vi "Codec_CMD_25.vi"(8 "error in (no error)":errorcluster, 10 "AskCMD25":T1={"STATION"="H/P", "RACK"="1", "DUT"="1"}, 11 "SecureMqttCodec in":refnum<class "SecureMqttCodec.lvclass">) -> (0 "error out":errorcluster, 2 "<JSON>":string="{\r  \"CMD\": 25,\r  \"CONTENT\": [\r    {\r      \"DUT\": \"1\",\r      \"RACK\": \"1\",\r      \"STATION\": \"H/P\"\r    }\r  ],\r  \"ERRCODE\": \"\",\r  \"ERRMSG\": \"\",\r  \"FROM\": \"845CF3525B43\",\r  \"ID\": \"BEEA132C-7671-42B7-B8AF-0AE4588F97BB\",\r  \"STATUS\": \"\",\r  \"TIMESTAMP\": 1759592435,\r  \"TO\": \"\"\r}", 3 "SecureMqttCodec out":refnum<class "SecureMqttCodec.lvclass">)   [LabVIEW 2020, in "SecureMqttCodec.lvclass"]
uses:
  SecureMqttCodec.lvclass
  TestMQTT/Ctrl/ReplyCMD25.ctl
  SecureMqttCodec.lvclass/SecureMqttCodec.ctl
  <vilib>/addons/JSON API/JSON Value/Set from JSON string.vi
  <vilib>/addons/JSON API/JSON Scalar/JSON Scalar.lvclass
  C:/Program Files/National Instruments/LabVIEW 2020/vi.lib/addons/JSON API/JSON Value/JSON Value.lvclass
  <vilib>/addons/JSON API/JSON Array/JSON Array.lvclass
  <vilib>/addons/JSON API/JSON Scalar/Set U32.vi
  <vilib>/addons/JSON API/JSON Array/Set JSON Array.vi
  <vilib>/addons/JSON API/JSON Value/Get as JSON string (pretty).vi
  <vilib>/addons/JSON API/JSON Value/JSON Value.lvclass
  <vilib>/addons/JSON API/Get Polymorphic/JSON GetSet.lvlib
  <vilib>/addons/JSON API/JSON Object/JSON Object.lvclass
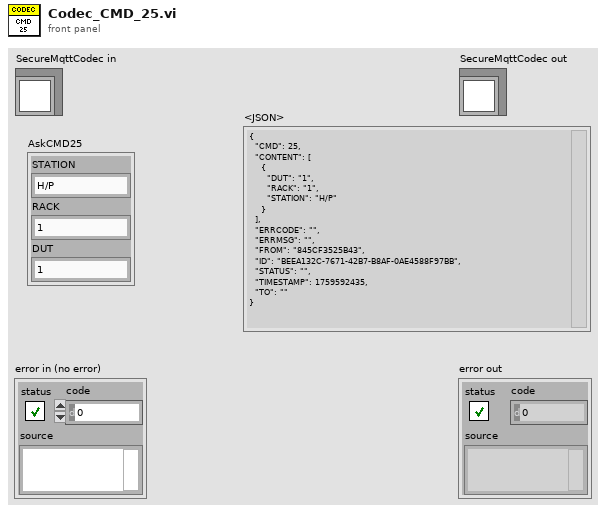
[diagram p1: front panel]
types:
  T1 = typedef "ReplyCMD25.ctl" = cluster{"STATION":string, "RACK":string, "DUT":string}
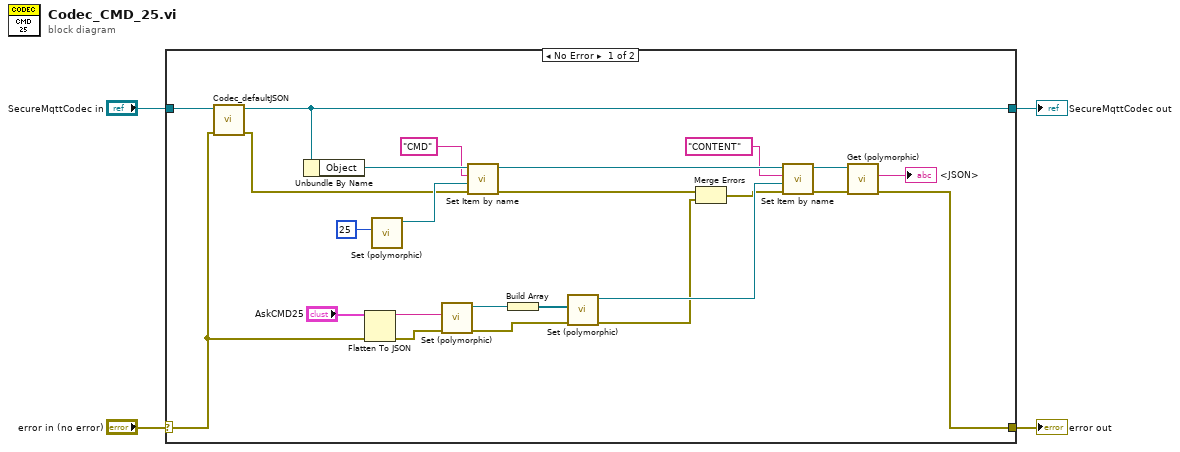
[diagram p0: block diagram]
diagram:
  n1 = case shown="No Error" "error in (no error)" {
    selector: "error in (no error)" -> [w8 w30]
    tunnel: [w24 w30] -> w3
    tunnel: [w16 w29] -> w1
    tunnel: "SecureMqttCodec in" -> [w28 w29]
    frame No Error {
      n2 = call "Codec_defaultJSON.vi"("error in (no error)"=w8, "SecureMqttCodec in"=w28) -> ("error out"=w15:errorcluster, "SecureMqttCodec out"=w16:refnum<class "SecureMqttCodec.lvclass">)  [unwired: 8 in]
      n3 = Unbundle By Name(w16) -> ("Object"=w27:refnum<class "JSON Value.lvclass">)
      n4 = Flatten To JSON(anything="AskCMD25", error in (no error)=w8) -> (JSON string=w10:string, 11:w9:errorcluster)  [unwired: 1 in]
      n5 = call-poly <vilib>:"Set (polymorphic).vi"("Numeric"=u32 25) -> ("JSON Scalar out"=w25:refnum<class "JSON Scalar.lvclass">)  [unwired: 9 in, 1 out]
      n6 = call-poly <vilib>:"Set (polymorphic).vi"("error in (no error)"=w9, "JSON stream"=w10) -> ("error out"=w7:errorcluster, "JSON Value out"=w12:refnum<class "JSON Value.lvclass">)  [unwired: 7 in, 1 out]
      n7 = call-dynamic "Set Item by name.vi"("error in (no error)"=w15, "Value"=w25, "name"="CMD", "JSON Value In"=w27) -> ("error out"=w20:errorcluster, "JSON Value Out"=w22:refnum<class "JSON Value.lvclass">)  [unwired: 5 in, 1 out]
      n8 = Build Array(w12) -> (w11:refnum<class "JSON Value.lvclass">[])
      n9 = call-poly <vilib>:"Set (polymorphic).vi"("error in (no error)"=w7, "Array"=w11) -> ("error out"=w5:errorcluster, "JSON Array out"=w18:refnum<class "JSON Array.lvclass">)  [unwired: 8 in]
      n10 = Merge Errors(w20, w5) -> (w6:errorcluster)
      n11 = call-dynamic "Set Item by name.vi"("error in (no error)"=w6, "Value"=w18, "name"="CONTENT", "JSON Value In"=w22) -> ("error out"=w19:errorcluster, "JSON Value Out"=w21:refnum<class "JSON Value.lvclass">)  [unwired: 5 in, 1 out]
      n12 = call-poly <vilib>:"Get (polymorphic).vi"("error in (no error)"=w19, "JSON Value in"=w21) -> ("error out"=w24:errorcluster, "<JSON>"=→"<JSON>":string)  [unwired: 8 in]
    }
    frame Error {
    }
  }
  "error out" <- w3
  "SecureMqttCodec out" <- w1
